vi "Destroy Shared Data DVR.vi"(8 "error in (no error)":errorcluster, 11 "Shared Data DVR":T2) -> (0 "error out":errorcluster, 3 "shared data":T1)   [LabVIEW 2017, in "DSF System Explorer.lvlib"]
uses:
  DSF System Explorer.lvlib
  shared data ref.ctl
  shared data.ctl
  DSF Core.lvlibp/Classes/Configuration/Configuration Session.lvclass
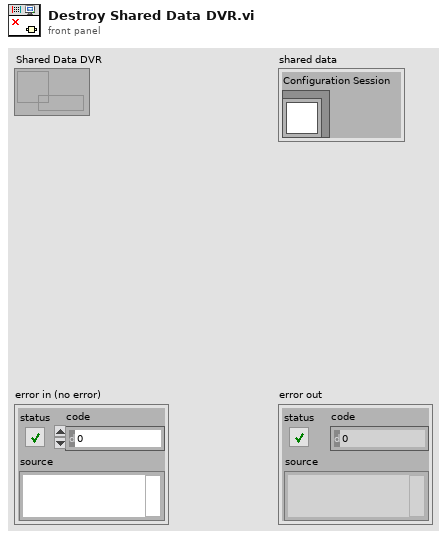
[diagram p1: front panel]
types:
  T1 = typedef "DSF System Explorer.lvlib/shared data.ctl" = cluster{"Configuration Session":refnum<class "Configuration Session.lvclass">}
  T2 = typedef "DSF System Explorer.lvlib/shared data ref.ctl" = refnum<data-value>
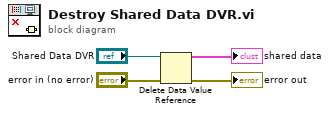
[diagram p0: block diagram]
diagram:
  n1 = Delete Data Value Reference(data value reference="Shared Data DVR", error in="error in (no error)") -> (data value=→"shared data":T1, error out=→"error out":errorcluster)
